vi "emi_NaN from extended array.vi"(7 "Float Array":ext[](array[numeric])) -> (8 "Float Array without NaN":ext[](array[numeric]))   [LabVIEW 2010]
doc: "Remove all nan values from an array for extended."
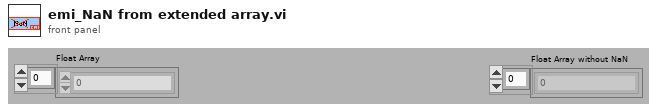
[diagram p1: front panel]
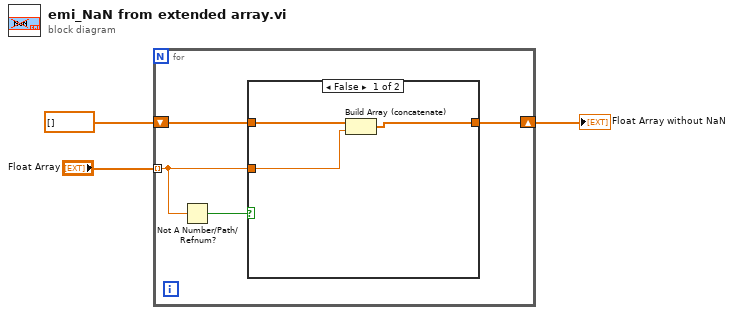
[diagram p0: block diagram]
diagram:
  n1 = for {
    tunnel: "Float Array" -> [w4] mode=indexing
    shift-right: [w5] -> w1
    shift-left: sgl[] [] ("Single Array") -> [w6]
    n2 = Not A Number/Path/Refnum?(number/path/refnum=w4) -> (NaN/Path/Refnum?=w7:bool)
    n3 = case shown="False" w7 {
      tunnel: w6 -> [w10 w11]
      tunnel: [w9 w11] -> w5
      tunnel: w4 -> [w8 _]
      frame False {
        n4 = Build Array (concatenate)(w10, w8) -> (w9:ext[])
      }
      frame True {
      }
    }
  }
  "Float Array without NaN" <- w1
